vi "find width.vi"(8 "Y Array":dbl[](array[numeric])=[0.0009018815801799904, 0.0013931365316602693, 0.002133156951295034, 0.0032377022502991927, 0.004871200099330652, 0.007264738716501479, 0.010739621970075901, 0.015737761397641555, 0.022860297871266706, 0.032915903447367105, 0.04698017615666683, 0.06646736595658473, 0.09321531302904634, 0.12958389288924066, 0.17856640257529716, 0.24391215453812712, 0.3302570535497631, 0.44325712761439334, 0.5897179132570423, 0.7777103500869236, 1.0166615614905485, 1.3174067832463723, 1.6921869952798436, 2.1545757987951584, 2.719319067800975, 3.4020721909719525, 4.219022567089984, 5.186389605399473, 6.319800870204833, 7.633551096245199, 9.139760297408586, 10.847457600757657, 12.7616280648146, 14.882269718142613, 17.20351639696773, 19.71288764652013, 22.3907290185756, 25.20990375734595, 28.135789609146435, 31.12662218868485, 34.13420930555854, 37.10501969670321, 39.98162598258847, 42.70445701436756, 45.21379102026229, 47.45190010928911, 49.36524067794993, 50.906574733674105, 52.03690527222507, 52.727115186698036, 52.95921360430245, 52.72711518669803, 52.03690527222506, 50.906574733674105, 49.36524067794991, 47.45190010928913, 45.21379102026226, 42.70445701436757, 39.98162598258844, 37.10501969670317, 34.13420930555854, 31.126622188684813, 28.135789609146414, 25.20990375734592, 22.390729018575584, 19.712887646520127, 17.203516396967714, 14.882269718142604, 12.761628064814579, 10.847457600757647, 9.139760297408593, 7.633551096245187, 6.319800870204827, 5.1863896053994605, 4.219022567089979, 3.4020721909719525, 2.7193190678009698, 2.1545757987951557, 1.6921869952798394, 1.3174067832463714, 1.0166615614905488, 0.7777103500869237, 0.5897179132570409, 0.4432571276143922, 0.33025705354976265, 0.24391215453812706, 0.17856640257529716, 0.12958389288924033, 0.09321531302904609, 0.06646736595658465, 0.04698017615666683, 0.032915903447367126, 0.02286029787126663, 0.0157377613976415, 0.0107396219700759, 0.007264738716501481, 0.004871200099330617, 0.0032377022502991814, 0.002133156951295026, 0.001393136531660269, 0.0009018815801799904], 11 "x Array":dbl[](array[numeric])=[-20.0, -19.6, -19.2, -18.8, -18.4, -18.0, -17.6, -17.2, -16.8, -16.4, -16.0, -15.6, -15.2, -14.8, -14.399999999999999, -14.0, -13.6, -13.2, -12.8, -12.399999999999999, -12.0, -11.6, -11.2, -10.799999999999999, -10.399999999999999, -10.0, -9.6, -9.2, -8.799999999999999, -8.399999999999999, -8.0, -7.6, -7.199999999999999, -6.799999999999999, -6.399999999999999, -6.0, -5.6, -5.199999999999999, -4.799999999999999, -4.399999999999999, -4.0, -3.599999999999998, -3.1999999999999993, -2.8000000000000007, -2.3999999999999986, -2.0, -1.5999999999999979, -1.1999999999999993, -0.7999999999999972, -0.3999999999999986, 0.0, 0.40000000000000213, 0.8000000000000007, 1.2000000000000028, 1.6000000000000014, 2.0, 2.400000000000002, 2.8000000000000007, 3.200000000000003, 3.6000000000000014, 4.0, 4.400000000000002, 4.800000000000001, 5.200000000000003, 5.600000000000001, 6.0, 6.400000000000002, 6.800000000000001, 7.200000000000003, 7.600000000000001, 8.0, 8.400000000000002, 8.8, 9.200000000000003, 9.600000000000001, 10.0, 10.400000000000002, 10.8, 11.200000000000003, 11.600000000000001, 12.0, 12.399999999999999, 12.800000000000004, 13.200000000000003, 13.600000000000001, 14.0, 14.399999999999999, 14.800000000000004, 15.200000000000003, 15.600000000000001, 16.0, 16.4, 16.800000000000004, 17.200000000000003, 17.6, 18.0, 18.400000000000006, 18.800000000000004, 19.200000000000003, 19.6, 20.0]) -> (0 "t2":dbl, 1 "t1":dbl, 3 "delt t":dbl=10.052835931648131)   [LabVIEW 2011]
panel:
  out "graph":cluster{"1D Array output":dbl[], dbl[]}(graph)={"1D Array output"=[-20.0, -19.6, -19.2, -18.8, -18.4, -18.0, -17.6, -17.2, -16.8, -16.4, -16.0, -15.6, -15.2, -14.8, -14.399999999999999, -14.0, -13.6, -13.2, -12.8, -12.399999999999999, -12.0, -11.6, -11.2, -10.799999999999999, -10.399999999999999, -10.0, -9.6, -9.2, -8.799999999999999, -8.399999999999999, -8.0, -7.6, -7.199999999999999, -6.799999999999999, -6.399999999999999, -6.0, -5.6, -5.199999999999999, -4.799999999999999, -4.399999999999999, -4.0, -3.599999999999998, -3.1999999999999993, -2.8000000000000007, -2.3999999999999986, -2.0, -1.5999999999999979, -1.1999999999999993, -0.7999999999999972, -0.3999999999999986, 0.0, 0.40000000000000213, 0.8000000000000007, 1.2000000000000028, 1.6000000000000014, 2.0, 2.400000000000002, 2.8000000000000007, 3.200000000000003, 3.6000000000000014, 4.0, 4.400000000000002, 4.800000000000001, 5.200000000000003, 5.600000000000001, 6.0, 6.400000000000002, 6.800000000000001, 7.200000000000003, 7.600000000000001, 8.0, 8.400000000000002, 8.8, 9.200000000000003, 9.600000000000001, 10.0, 10.400000000000002, 10.8, 11.200000000000003, 11.600000000000001, 12.0, 12.399999999999999, 12.800000000000004, 13.200000000000003, 13.600000000000001, 14.0, 14.399999999999999, 14.800000000000004, 15.200000000000003, 15.600000000000001, 16.0, 16.4, 16.800000000000004, 17.200000000000003, 17.6, 18.0, 18.400000000000006, 18.800000000000004, 19.200000000000003, 19.6, 20.0], [0.0009018815801799904, 0.0013931365316602693, 0.002133156951295034, 0.0032377022502991927, 0.004871200099330652, 0.007264738716501479, 0.010739621970075901, 0.015737761397641555, 0.022860297871266706, 0.032915903447367105, 0.04698017615666683, 0.06646736595658473, 0.09321531302904634, 0.12958389288924066, 0.17856640257529716, 0.24391215453812712, 0.3302570535497631, 0.44325712761439334, 0.5897179132570423, 0.7777103500869236, 1.0166615614905485, 1.3174067832463723, 1.6921869952798436, 2.1545757987951584, 2.719319067800975, 3.4020721909719525, 4.219022567089984, 5.186389605399473, 6.319800870204833, 7.633551096245199, 9.139760297408586, 10.847457600757657, 12.7616280648146, 14.882269718142613, 17.20351639696773, 19.71288764652013, 22.3907290185756, 25.20990375734595, 28.135789609146435, 31.12662218868485, 34.13420930555854, 37.10501969670321, 39.98162598258847, 42.70445701436756, 45.21379102026229, 47.45190010928911, 49.36524067794993, 50.906574733674105, 52.03690527222507, 52.727115186698036, 52.95921360430245, 52.72711518669803, 52.03690527222506, 50.906574733674105, 49.36524067794991, 47.45190010928913, 45.21379102026226, 42.70445701436757, 39.98162598258844, 37.10501969670317, 34.13420930555854, 31.126622188684813, 28.135789609146414, 25.20990375734592, 22.390729018575584, 19.712887646520127, 17.203516396967714, 14.882269718142604, 12.761628064814579, 10.847457600757647, 9.139760297408593, 7.633551096245187, 6.319800870204827, 5.1863896053994605, 4.219022567089979, 3.4020721909719525, 2.7193190678009698, 2.1545757987951557, 1.6921869952798394, 1.3174067832463714, 1.0166615614905488, 0.7777103500869237, 0.5897179132570409, 0.4432571276143922, 0.33025705354976265, 0.24391215453812706, 0.17856640257529716, 0.12958389288924033, 0.09321531302904609, 0.06646736595658465, 0.04698017615666683, 0.032915903447367126, 0.02286029787126663, 0.0157377613976415, 0.0107396219700759, 0.007264738716501481, 0.004871200099330617, 0.0032377022502991814, 0.002133156951295026, 0.001393136531660269, 0.0009018815801799904]}
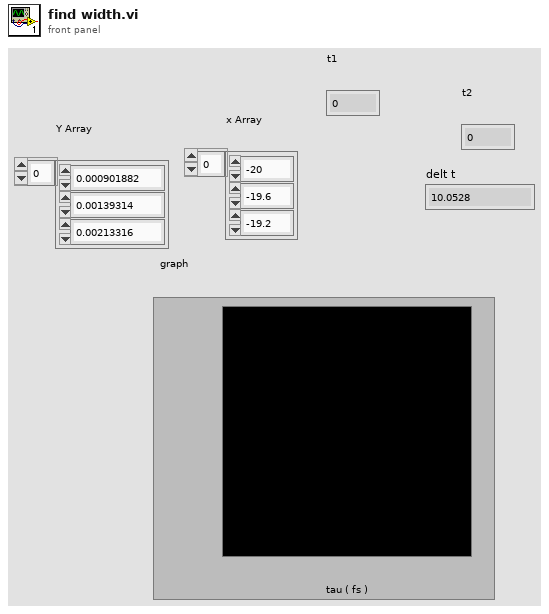
[diagram p1: front panel]
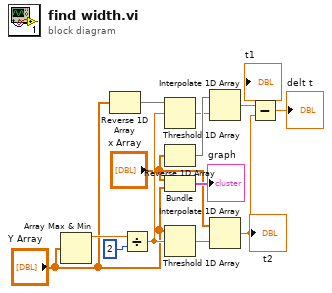
[diagram p0: block diagram]
diagram:
  n1 = Array Max & Min(array="Y Array") -> (max value=w10:dbl)  [unwired: 3 out]
  n2 = Reverse 1D Array(array="Y Array") -> (reversed array=w8:dbl[])
  n3 = Divide(x=w10, y=2) -> (x/y=w7:dbl)
  n4 = Threshold 1D Array(2:w7, 3:w8) -> (0:w6:dbl)  [unwired: 1 in]
  n5 = Reverse 1D Array(array="x Array") -> (reversed array=w9:dbl[])
  n6 = Bundle("x Array"="x Array", "Y Array"="Y Array") -> (→"graph":cluster{"x Array":dbl[], "Y Array":dbl[]})  [unwired: 1 in]
  n7 = Threshold 1D Array(2:w7, 3:"Y Array") -> (0:w11:dbl)  [unwired: 1 in]
  n8 = Interpolate 1D Array(1:w6, 2:w9) -> (0:w5:dbl)
  "t1" <- w5
  n9 = Interpolate 1D Array(1:w11, 2:"x Array") -> (0:w4:dbl)
  "t2" <- w4
  n10 = Subtract(x=w5, y=w4) -> (x-y=→"delt t":dbl)
